vi "Connection to String.vi"(11 "Connection":T1) -> (3 "String":string)   [LabVIEW 2017, in "Switch Scripting.lvlib"]
uses:
  Switch Scripting.lvlib
  Routing Channel/Connection.ctl
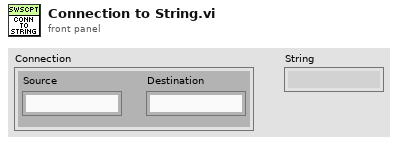
[diagram p1: front panel]
types:
  T1 = typedef "Switch Scripting.lvlib/Connection.ctl" = cluster{"Source":string, "Destination":string}
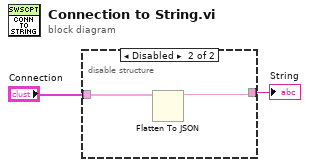
[diagram p0: block diagram]
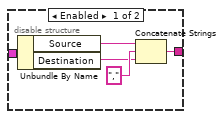
[diagram p2: hidden frame]
diagram:
  n1 = disable-structure shown="Disabled" {
    disable-tunnel: [w7 w8] -> w2
    disable-tunnel: "Connection" -> [w3 w9]
    frame Enabled {
      n2 = Unbundle By Name(w3) -> ("Source"=w5:string, "Destination"=w4:string)
      n3 = Concatenate Strings(w5, "," ("string"), w4) -> (w7:string)
    }
    frame Disabled {
      n4 = Flatten To JSON(anything=w9) -> (JSON string=w8:string)  [unwired: 2 in, 1 out]
    }
  }
  "String" <- w2
